vi "Sliding DAQ.vi"() -> ()   [LabVIEW 2021]
uses:
  <vilib>/Simulation/Scripting/Companion Diagram/SimConfigNode/SimParams.ctl
  <vilib>/Simulation/Scripting/Companion Diagram/SimConfigNode/_simSolvers.ctl
  <vilib>/Simulation/Implementation/Shared/SIMSCR Execution Mode.ctl
  <vilib>/Simulation/Param Hierarchy/Typedefs/SIMPH Param Control Actions.ctl
  <vilib>/Simulation/Implementation/Shared/NILVSim_ParamChanged.vi
  <vilib>/Simulation/Implementation/Shared/NILVSIM_BeginStep.vi
  <vilib>/Simulation/DataSources/Implementation/NILVSim Step.llb/SIM Step (scalar).vi
  <vilib>/Simulation/ContinuousLinear/Implementation/NILVSim Derivative.llb/SIM derivative (scalar).vi
  <vilib>/Simulation/SignalArithmetic/Implementation/NILVSim Gain.llb/SIM Gain (scalar).vi
  <vilib>/Simulation/SignalArithmetic/Implementation/NILVSim Gain.llb/SIM Gain (vector).vi
  <vilib>/Simulation/ContinuousLinear/Implementation/NILVSim Derivative.llb/SIM derivative (vector).vi
  <vilib>/Simulation/Nonlinear/Implementation/NILVSim Saturation.llb/SIM Saturation (vector).vi
  <vilib>/Simulation/Implementation/Shared/NILVSim_Manager.vi
  <vilib>/Utility/error.llb/Clear Errors.vi
  <vilib>/Simulation/Implementation/Shared/NILVSim_FinalizeModel.vi
  <vilib>/Simulation/Implementation/Shared/SIM Unbundle Sim Info.vi
  <vilib>/Simulation/Implementation/Shared/NILVSim_Initialize.vi
  <vilib>/Simulation/Utility/Implementation/NILVSim Get Time and IsAcceptedStep.vi
  <vilib>/Simulation/Implementation/Shared/SIMSH Read Queue.vi
  <vilib>/Simulation/Implementation/Shared/NILVSim_GetModelError.vi
  <vilib>/Simulation/Implementation/Shared/SIM Bundle Sim Info.vi
  <vilib>/Simulation/Scripting/Companion Diagram/SimConfigNode/SimDog.xnode
  <vilib>/Simulation/Implementation/XNodeFramework/SimXNode/SimX.xnode
  <vilib>/Simulation/Implementation/Shared/NI_SIM_Implementation.lvlib
panel:
  out "Graph 2":waveform(dbl)[](graph)
  out "Graph":waveform(dbl)[](graph)
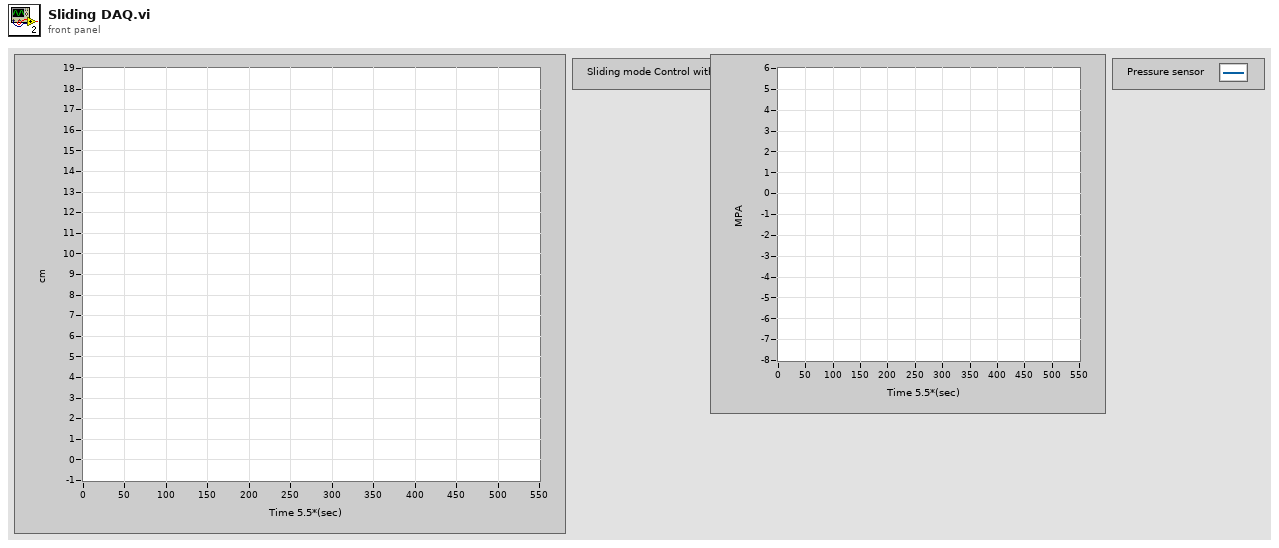
[diagram p1: front panel]
types:
  T1 = typedef "SIMSCR Execution Mode.ctl" = enum16{"Simulate to Completion", "Single Time-Step Simulation (Fixed Step Only)"}
  T2 = typedef "SIMPH Param Control Actions.ctl" = enum16{"get params", "set params"}
  T3 = typedef "SimParams.ctl" = cluster{"Initial Time (s)":dbl, "Final Time (s)":dbl, "Step Size (s)":dbl, "ODE Solver":T4, "Minimum Step Size (s)":dbl, "Maximum Step Size (s)":dbl, "Relative Tolerance":dbl, "Absolute Tolerance":dbl, "Software Timing":bool, "Initial Step Size (s)":dbl, "Automatic Fixed Step Size?":bool, "Automatic Discrete Step Size?":bool, "Discrete Step Size (s)":dbl, "Calculate using Time Step":bool, "Solver Wired?":bool, "Prev.Frm.Expected End":u64, "Prev.Frm.Actual End":u64, "Prev.Frm.Finished Late?":bool, "Prev.Iter.Expected End":u64, "Prev.Iter.Actual End":u64, "Prev.Iter.Finished Late?":bool, "Expected Iteration Start":u64, "Actual Iteration Start":u64, "Expected Frame Start":u64, "Actual Frame Start":u64, "Source Name":string, "Name":string, "Period":i64, "Deadline":i64, "Offset":i64, "Start":i64, "Priority":i32, "Timeout":i32, "Processor":i32, "Mode":enum32{"No Change", "Process missed periods, maintain original phase", "Discard missed periods, maintain original phase", "Process missed periods, ignore original phase", "Discard missed periods, ignore original phase"}, "Wakeup reason":enum32{"Normal", "Aborted", "Asynchronous wakeup", "Timing source error", "Timed loop error", "Timeout"}, "Error":errorcluster, "Source Type":string, "Secondary Source Type":string, "Global End Time":u64, "Global Start Time":u64, "Full Solver Reset":bool, "Execution Mode":T1, "Nan/Inf Check":bool, "Custom Solver Library":string, "Solver Is Variable":bool, "custom solver name":string, "Signal Collection Decimation":u32}
  T4 = typedef "_simSolvers.ctl" = enum16{"Runge-Kutta 1 (Euler)", "Runge-Kutta 2", "Runge-Kutta 3", "Runge-Kutta 4", "Runge-Kutta 23 (variable)", "Runge-Kutta 45 (variable)", "BDF (variable)", "Adams-Moulton (variable)", "Rosenbrock (variable)", "Discrete States Only", "SDIRK 4 (variable)", "Radau 5 (variable)", "Radau 9 (variable)", "Radau 13 (variable)", "Radau [Variable Order] (variable)", "Gear's Method (variable)", "Linearizer", "State Query", "Trim Eval", "Custom Solver"}
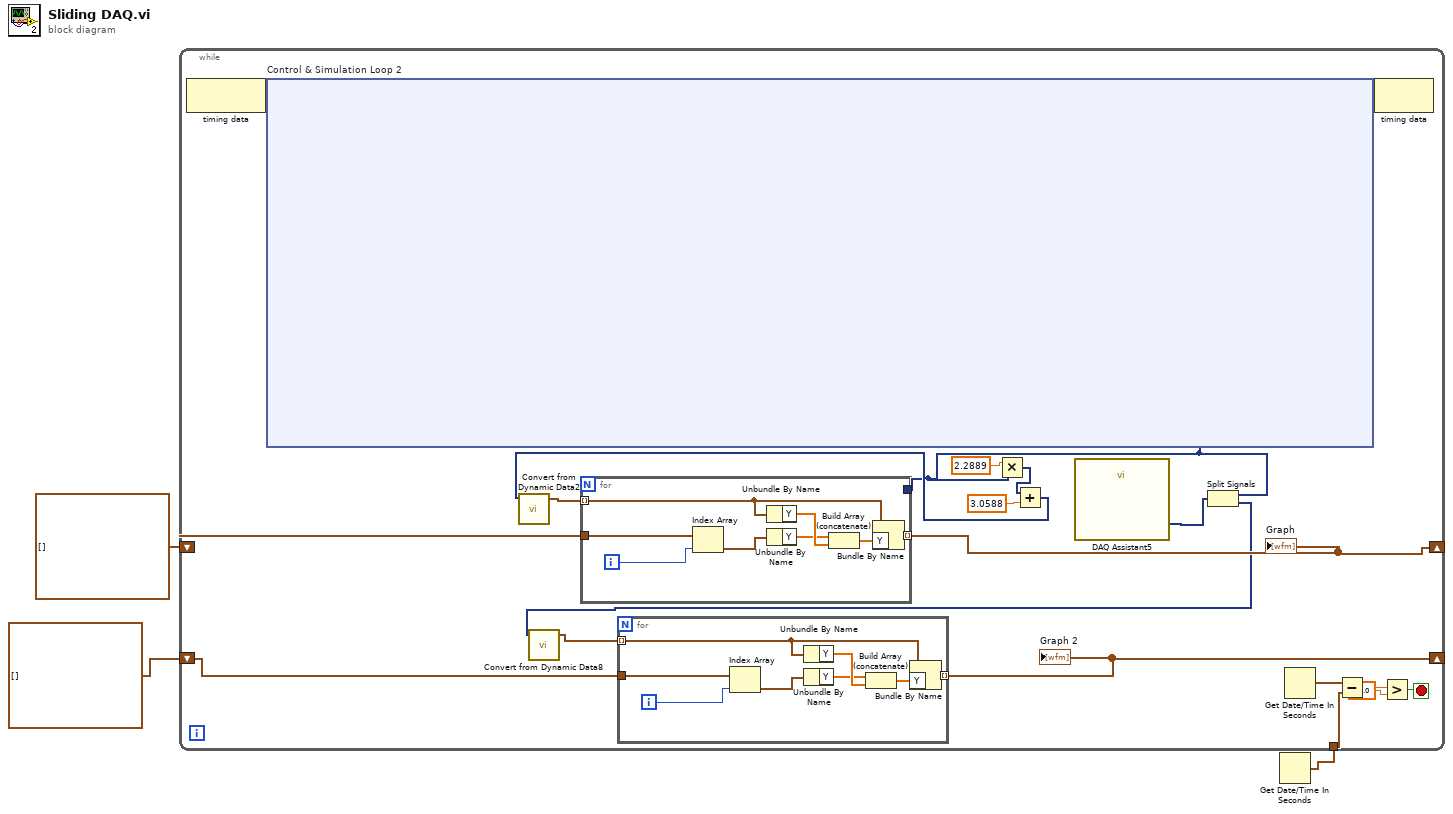
[diagram p0: block diagram]
diagram:
  n1 = Get Date/Time In Seconds() -> (seconds since 1Jan1904=w2:timestamp)
  n2 = while {
    shift-right: [w19] -> _
    shift-left: waveform(dbl)[] [] -> [w21]
    tunnel: w2 -> [w17]
    shift-right: [w8] -> _
    shift-left: waveform(dbl)[] [] -> [w9]
    stop <- w14 stop-if-true
    n3 = node-c288() -> (w23:variant)  [unwired: 1 in]
    n4 = call "DAQ Assistant5"() -> ("data"=w6:dynamicdata)  [unwired: 17 in, 2 out]
    n5 = Split Signals(w6) -> (w4:dynamicdata, w5:dynamicdata)  [unwired: 2 in]
    n6 = node-c254 "Control & Simulation Loop 2"(w23, w4) -> (w22:variant)
    n7 = call "Convert from Dynamic Data8"("Dynamic Data Type"=w5) -> ("Array of Waveform"=w7:waveform(dbl)[])  [unwired: 3 in]
    n8 = for {
      tunnel: w9 -> [w26]
      tunnel: w7 -> [w24] mode=indexing
      tunnel: [w25] -> w8 mode=indexing
      i -> [w27]
      n9 = Index Array(array=w26, index=w27) -> (element=w31:waveform(dbl))
      n10 = Unbundle By Name(w24) -> ("Y"=w30:dbl[])
      n11 = Unbundle By Name(w31) -> ("Y"=w28:dbl[])
      n12 = Build Array (concatenate)(w28, w30) -> (w29:dbl[])
      n13 = Bundle By Name(cluster=w24, "Y"=w29) -> (w25:waveform(dbl))
    }
    "Graph 2" <- w8
    n14 = Multiply(x=2.2889 ("y"), y=w4) -> (x*y=w11:dynamicdata)
    n15 = Add(x=w11, y=3.0588) -> (x+y=w10:dynamicdata)
    n16 = call "Convert from Dynamic Data2"("Dynamic Data Type"=w10) -> ("Array of Waveform"=w20:waveform(dbl)[])  [unwired: 3 in]
    n17 = for {
      tunnel: w21 -> [w34]
      tunnel: w20 -> [w32] mode=indexing
      tunnel: [w33] -> w19 mode=indexing
      tunnel: w4 -> [_]
      i -> [w35]
      n18 = Index Array(array=w34, index=w35) -> (element=w39:waveform(dbl))
      n19 = Unbundle By Name(w32) -> ("Y"=w38:dbl[])
      n20 = Unbundle By Name(w39) -> ("Y"=w36:dbl[])
      n21 = Build Array (concatenate)(w36, w38) -> (w37:dbl[])
      n22 = Bundle By Name(cluster=w32, "Y"=w37) -> (w33:waveform(dbl))
    }
    "Graph" <- w19
    n23 = Get Date/Time In Seconds() -> (seconds since 1Jan1904=w18:timestamp)
    n24 = Subtract(x=w18, y=w17) -> (x-y=w16:dbl)
    n25 = node-c288(w22) -> ()  [unwired: 1 out]
    n26 = Greater?(x=w16, y=100.0) -> (0:w14:bool)
  }
